vi "Cleanup.vi"(8 "error in (no error)":errorcluster, 11 "AppDetailPanel in":refnum<class "AppDetailPanel.lvclass">) -> (0 "error out":errorcluster)   [LabVIEW 2020, in "PicoG-App.lvlib" / "AppDetailPanel.lvclass"]
uses:
  AppDetailPanel.lvclass
  AppDetailPanel.lvclass/AppDetailPanel.ctl
  <vilib>/IlluminatedG/IG OOPanel/OOPanel/Panel/Panel.lvclass
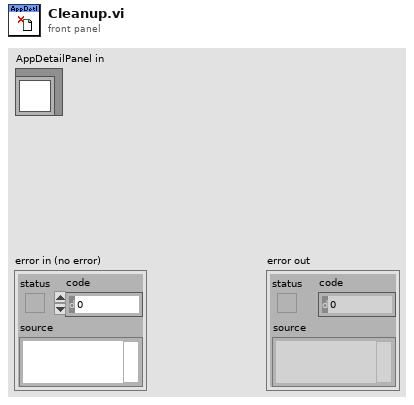
[diagram p1: front panel]
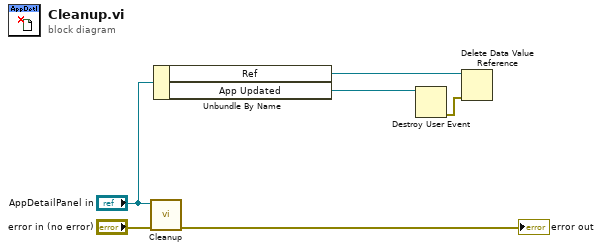
[diagram p0: block diagram]
diagram:
  n1 = call-parent "Cleanup.vi"("error in (no error)"="error in (no error)", "Panel in"="AppDetailPanel in") -> ("error out"=→"error out":errorcluster)  [unwired: 9 in]
  n2 = Unbundle By Name("AppDetailPanel in") -> ("Ref"=w2:refnum<data-value>, "App Updated"=w3:refnum<user-event>)
  n3 = Destroy User Event(user event=w3) -> (error out=w1:errorcluster)  [unwired: 1 in]
  n4 = Delete Data Value Reference(data value reference=w2, error in=w1) -> ()  [unwired: 2 out]
